vi "WebRes_GetOnlineData.vi"(7 "LabVIEW Web Service Request":refnum<class "Web Request.lvclass">) -> ()   [LabVIEW 2018]
doc: "get System online data from DVR and transmit this over WebService"
uses:
  <vilib>/wsapi/Web Request.lvclass
  _MonSys_LIB/OnlineData.ctl
  _MonSys_LIB/OnlineData_State.ctl
  MonSys_Server_Sources/MonSys_Server_Actor/typedefs/OnlineData_HandleDVR_func.ctl
  MonSys_Server_Sources/MonSys_Server_Actor/MonSys_Server_Actor.lvclass
  _MonSys_LIB/_MonSys_LIB.lvlib
panel:
  out "Sended_OnlineData":T1={"Online"=TRUE, "Info"="", "OnlineData_State"=0} {"OnlineData_State" items=["Idle", "Manually", "Automatic"]}
  out "WebService error":errorcluster
  out "DVR error":errorcluster
  out "First Call?":bool
  # "Use the Web Service Request input terminal to call the VIs on the Web Services palette. Do not remove it from the connector pane unless you don't need access to the palette."
  # "Each additional control wired to the connector pane will \nbe available as an input in the URL. To include an indicator\n in terminal-mode output (the default setting), it must also \nbe wired to the connector pane."
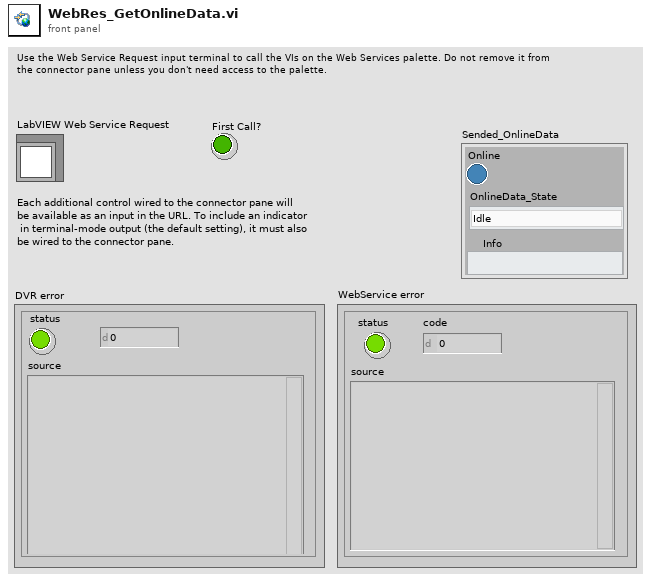
[diagram p1: front panel]
types:
  T1 = typedef "_MonSys_LIB.lvlib/OnlineData.ctl" = cluster{"Online":bool, "Info":string, "OnlineData_State":T2}
  T2 = typedef "_MonSys_LIB.lvlib/OnlineData_State.ctl" = u16
  T3 = typedef "OnlineData_HandleDVR_func.ctl" = enum16{"create", "get", "close"}
  T4 = typedef "MonSys_LIB.lvlib/OnlineData.ctl" = cluster{"Online":bool, "Info":string, "OnlineData_State":T5}
  T5 = typedef "MonSys_LIB.lvlib/OnlineData_State.ctl" = u16
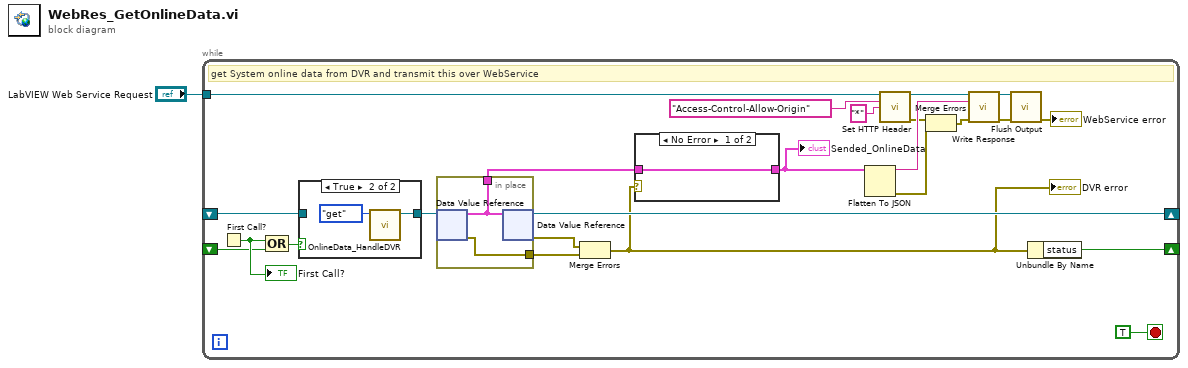
[diagram p0: block diagram]
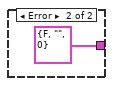
[diagram p2: hidden frame]
diagram:
  n1 = while {
    tunnel: "LabVIEW Web Service Request" -> [w21]
    shift-right: [w13] -> _
    shift-left: _ -> [w16]
    shift-right: [w12] -> _
    shift-left: _ -> [w11]
    stop <- TRUE stop-if-true
    # "get System online data from DVR and transmit this over WebService"
    n2 = First Call?() -> (First Call?: T/F=w17:bool)
    "First Call?" <- w17
    n3 = Compound Arithmetic op=OR(w17, w11) -> (w9:bool)
    n4 = case shown="True" w9 {
      tunnel: [w28 w30] -> w10
      tunnel: w16 -> [w28 _]
      frame False {
      }
      frame True {
        n5 = call "OnlineData_HandleDVR.vi"("func"=OnlineData_HandleDVR_func."get") -> ("DVR_OUT"=w30:refnum<data-value>)  [unwired: 9 in, 1 out]
      }
    }
    n6 = in-place {
      in-place-border: [w31] -> w3
      in-place-border: [w32] -> w14
      n7 = in-place-dvr #1(w10) -> (w31:T4, w32:errorcluster)
      n8 = in-place-dvr #1(w31) -> (w13:refnum<data-value>, w15:errorcluster)
    }
    n9 = Merge Errors(w15, w14) -> (w8:errorcluster)
    "DVR error" <- w8
    n10 = case shown="No Error" w8 {
      tunnel: [w26 T1 {"Online"=FALSE, "Info"="", "OnlineData_State"=0}] -> w2
      tunnel: w3 -> [w26 _]
      frame No Error {
      }
      frame Error {
      }
    }
    "Sended_OnlineData" <- w2
    n11 = Flatten To JSON(anything=w2) -> (JSON string=w25:string, 11:w6:errorcluster)  [unwired: 2 in]
    n12 = call <vilib>:"Set HTTP Header.vi"("LabVIEW Web Service Request"=w21, "header"="Access-Control-Allow-Origin", "header value"="*") -> ("LabVIEW Web Service Request out"=w22:refnum<class "Web Request.lvclass">, "error out"=w4:errorcluster)  [unwired: 11 in]
    n13 = Merge Errors(w4, w6) -> (w5:errorcluster)
    n14 = call <vilib>:"Write Response.vi"("LabVIEW Web Service Request"=w22, "response string"=w25, "error in (no error)"=w5) -> ("LabVIEW Web Service Request out"=w24:refnum<class "Web Request.lvclass">, "error out"=w23:errorcluster)  [unwired: 11 in]
    n15 = call <vilib>:"Flush Output.vi"("LabVIEW Web Service Request"=w24, "error in (no error)"=w23) -> ("error out"=→"WebService error":errorcluster)  [unwired: 12 in, 1 out]
    n16 = Unbundle By Name(w8) -> ("status"=w12:bool)
  }
